vi "remoteControlTest.vi"() -> ()   [LabVIEW 2019]
uses:
  <vilib>/ReMiSYS/ReMiSYS_WSCbot-XS/SubVI/XS_F710.ctl
  <vilib>/ReMiSYS/ReMiSYS_WSCbot-XS/SubVI/XS_stick.ctl
  <vilib>/ReMiSYS/ReMiSYS_WSCbot-XS/SubVI/XS_gamepadF710.lvclass
  WSCbot_V3_Toolkit.lvlibp/WSCBOTV3_Toolkit/IO/LowLevel/PulseCounter.ctl
  <vilib>/Platform/TimedLoop/XDataNode/timing_clust.ctl
  <vilib>/Platform/TimedLoop/XDataNode/nitl_modes.ctl
  <vilib>/Platform/TimedLoop/XDataNode/wakeup.ctl
  WSCbot_V3_Toolkit.lvlibp/WSCBOTV3_Toolkit/IO/LowLevel/IO_Chanel_DIO.ctl
  <vilib>/platform/TimedLoop/XDataNode/XDataNode.xnode
  <vilib>/Platform/TimedLoop/XDataNode/XDNodeRunTimeDep.lvlib
  WSCbot_V3_Toolkit.lvlibp
panel:
  out "leftStick_Touch\nTimes":i8
  in  "High_array(mm)":dbl[](array[numeric])=[0.0, 113.0, 200.0, 300.0]
  out "Hight":i32
  out "Front/Back":bool
  out "F710 button info.rightStick":bool
  out "up":bool
  out "Car move (cm)":dbl
  out "Wheel move (cm)":dbl[](array[numeric])
  out "F710 button info.leftStick":bool
  out "F710 button info.B":bool
  out "F710 button info.X":bool
  out "F710 button info.A":bool
  out "F710 button info.Y":bool
  out "F710 button info.RB":bool
  out "F710 button info.LB":bool
  out "ini":bool
  out "reset":bool
  out "UD touch?":bool
  out "high":dbl
  out "turn touch?":bool
  out "angle":dbl
  out "speed":dbl
  out "Error Out":errorcluster
  in  "Stop Button":bool
  in  "error in (no error)":errorcluster
  in  "INPUT S/N":string="U16N121E"
  in  "VISA resource name":refnum<visa-resource-name>="USB0::0x046D::0xC21F::145C9E1C::RAW"
  out "Stop Output":bool
  out "StepmotorTarget(mm)":dbl
  out "AxisPosition":dbl
  out "SpeedArray":dbl[](array[numeric])
  out "F710":T1
  in  "maxSpeed":dbl=800.0 format="%#_13g"
  # "總高度300mm"
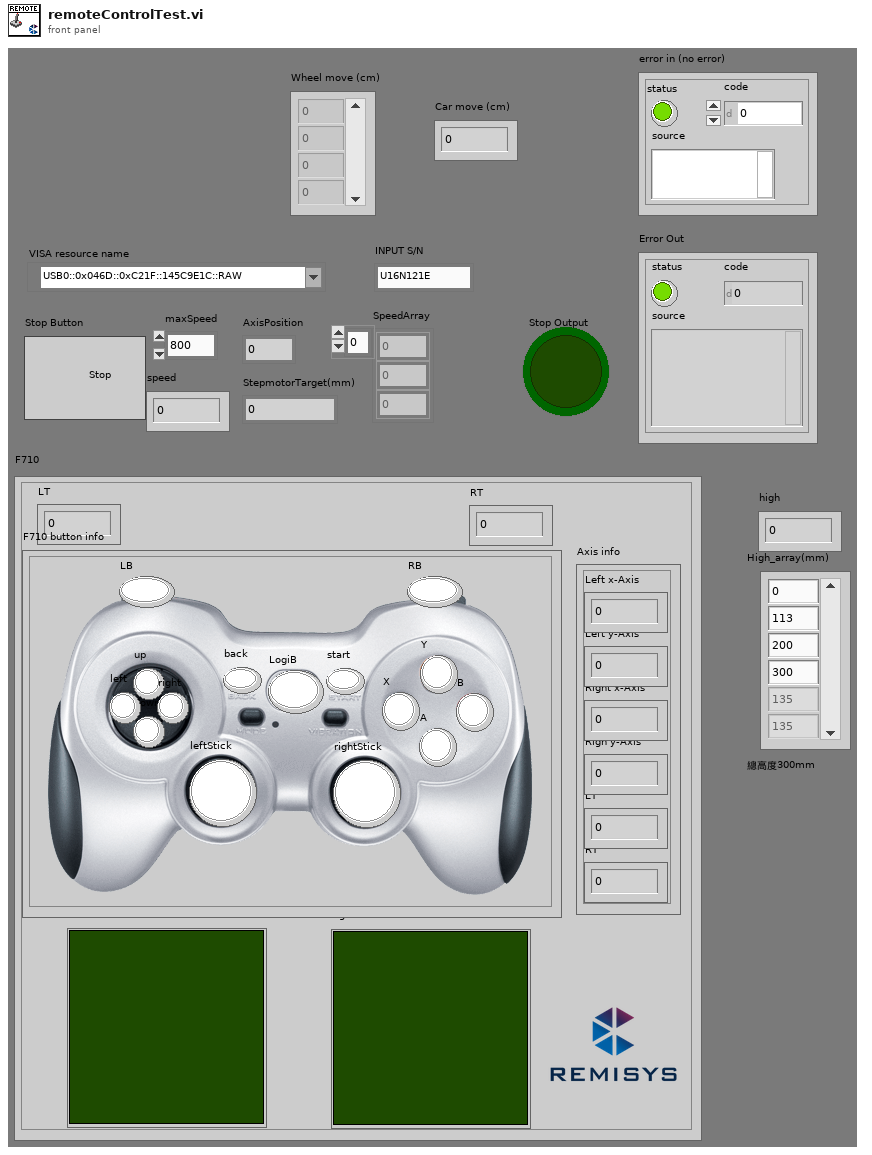
[diagram p1: front panel]
types:
  T1 = typedef "XS_F710.ctl" = cluster{"RT":u8, "LT":u8, "RightStick":T2, "LeftStick":T2, "Axis info":cluster{"Left x-Axis":i8, "Left y-Axis":i8, "Right x-Axis":i8, "Righ y-Axis":i8, "LT":u8, "RT":u8}, "F710 button info":cluster{"RB":bool, "LB":bool, "rightStick":bool, "leftStick":bool, "start":bool, "back":bool, "right":bool, "left":bool, "down":bool, "up":bool, "Y":bool, "X":bool, "B":bool, "A":bool, "LogiB":bool}}
  T2 = typedef "XS_stick.ctl" = cluster{"X":dbl, "Y":dbl}[]
  T3 = typedef "WSCbot_V3_Toolkit.lvlibp/PulseCounter.ctl" = enum16{"CH1", "CH2", "CH3", "CH4", "CH5"}
  T4 = typedef "WSCbot_V3_Toolkit.lvlibp/IO_Chanel_DIO.ctl" = enum16{"A/DIO9", "A/DIO10", "C/DIO0", "C/DIO1", "C/DIO2", "C/DIO3", "C/DIO4", "C/DIO5", "C/DIO6"}
  T5 = typedef "XDNodeRunTimeDep.lvlib/timing_clust.ctl" = cluster{"Expected End [f-1]":u64, "Actual End [f-1]":u64, "Finished Late? [f-1]":bool, "Expected End [i-1]":u64, "Actual End [i-1]":u64, "Finished Late? [i-1]":bool, "Expected Start [i]":u64, "Actual Start [i]":u64, "Expected Start [f]":u64, "Actual Start [f]":u64, "Source Name":string, "Structure Name":string, "Period":i64, "Deadline":i64, "Offset":i64, "Start":i64, "Priority":i32, "Timeout":i32, "Mode":T6, "Wakeup Reason":T7, "Error":errorcluster, "Source Type":string, "Secondary Source Type":string, "Global End Time":u64, "Global Start Time":u64, "Frame Duration":u64, "Iteration Duration":u64, "Assigned CPU":i32, "I/O Scan Engine Mode":u32}
  T6 = typedef "XDNodeRunTimeDep.lvlib/nitl_modes.ctl" = enum32{"No Change", "Process missed periods, maintain original phase", "Discard missed periods, maintain original phase", "Process missed periods, ignore original phase", "Discard missed periods, ignore original phase"}
  T7 = typedef "XDNodeRunTimeDep.lvlib/wakeup.ctl" = enum32{"Normal", "Aborted", "Asynchronous wakeup", "Timing source error", "Timed loop error", "Timeout"}
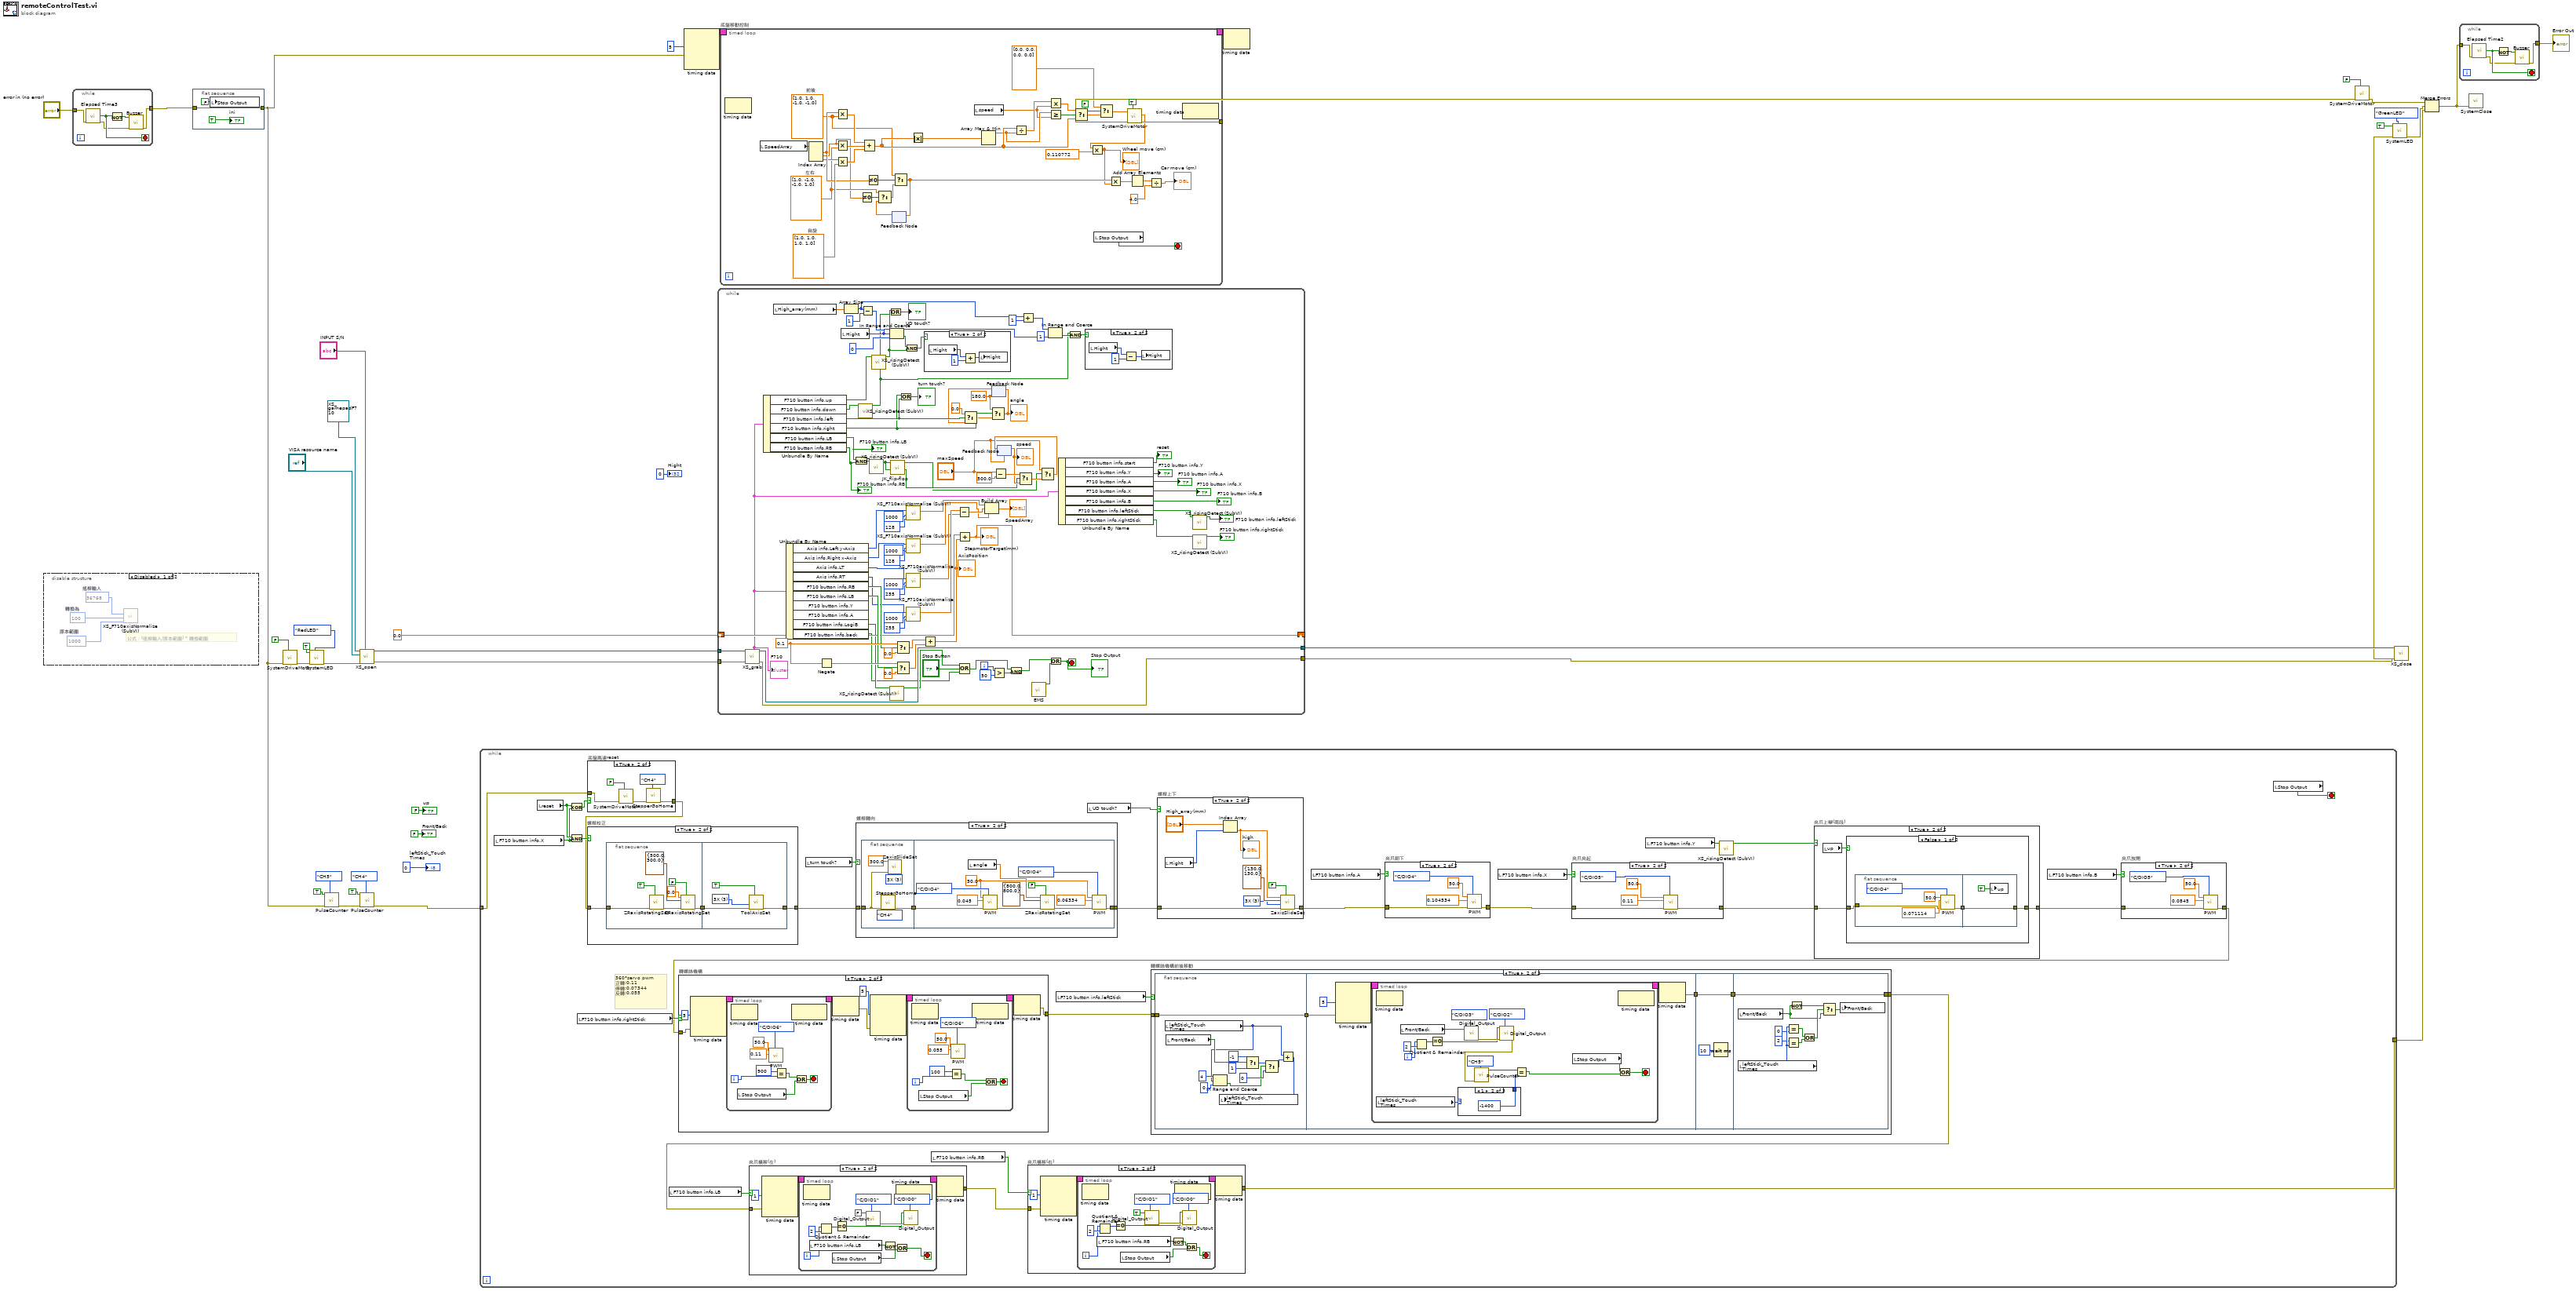
[diagram p0: block diagram]
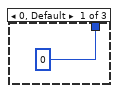
[diagram p5: hidden frame]
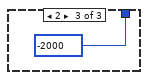
[diagram p6: hidden frame]
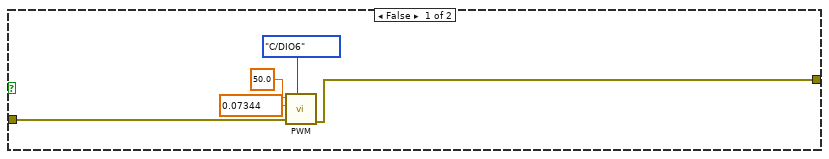
[diagram p7: hidden frame]
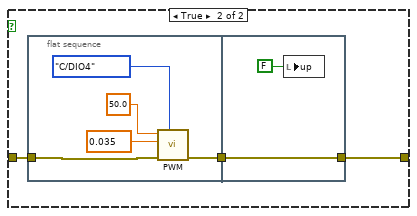
[diagram p12: hidden frame]
diagram:
  n1 = disable-structure shown="Disabled" {
    frame Disabled {
      w40 = 1000  # 原本範圍
      w41 = 100  # 轉換為
      w42 = 36768  # 搖桿輸入
      # "公式：(搖桿輸入/原本範圍) * 轉換範圍"
      n2 = call <vilib>:"XS_F710axisNormalize (SubVI).vi"("rawRange"=w40, "normalizeTo"=w41, "axisInput"=w42) -> ()  [unwired: 8 in, 1 out]
    }
    frame Enabled {
    }
  }
  n3 = while {
    tunnel: "error in (no error)" -> [w45]
    tunnel: [w43] -> w23
    stop <- w47 stop-if-true
    n4 = call "Elapsed Time3"("error in (no error)"=w45) -> ("Time has Elapsed"=w47:bool, "error out"=w44:errorcluster)  [unwired: 11 in, 6 out]
    n5 = Not(x=w47) -> (.not. x?=w46:bool)
    n6 = call "Buzzer.vi"("error in"=w44, "Set"=w46) -> ("error out"=w43:errorcluster)  [unwired: 9 in]
  }
  n7 = flat-sequence {
    tunnel: [w49] -> w7
    tunnel: w23 -> [w49]
    frame #0 {
      n8 = local write "Stop Output"(FALSE ("Stop Output")) -> ()
      "ini" <- TRUE
    }
  }
  n9 = call "SystemDriveMotor.vi"("Enable?"=FALSE, "error in"=w7) -> ("error out"=w19:errorcluster)  [unwired: 8 in, 1 out]
  n10 = call "SystemLED.vi"("SelectColor"=enum16{"RedLED", "GreenLED", "YellowLED"}."RedLED", "error in"=w19, "Set"=TRUE) -> ("error out"=w30:errorcluster)  [unwired: 8 in]
  n11 = call "PulseCounter.vi"("PulseCounterChanel"=PulseCounter."CH5", "error in"=w7, "Reset"=TRUE) -> ("error out"=w3:errorcluster)  [unwired: 7 in, 1 out]
  n12 = call <vilib>:"XS_open.vi"("INPUT S/N"="INPUT S/N", "error in (no error)"=w30, "VISA resource name"="VISA resource name", "gamepadF710 in"=refnum<class "XS_gamepadF710.lvclass"> refnum) -> ("error out"=w20:errorcluster, "gamepadF710 out"=w31:refnum<class "XS_gamepadF710.lvclass">)  [unwired: 6 in]
  n13 = call "PulseCounter.vi"("PulseCounterChanel"=PulseCounter."CH4", "error in"=w3, "Reset"=TRUE) -> ("error out"=w2:errorcluster)  [unwired: 7 in, 1 out]
  n14 = while {
    tunnel: w2 -> [w54]
    tunnel: [w57] -> w8
    stop <- w79 stop-if-true
    # "360°servo pwm\n正轉:0.11\n停轉:0.07344\n反轉:0.055"
    n15 = local read "F710 button info.X"() -> (w74:bool)
    n16 = local read "reset"() -> (w75:bool)
    n17 = Exclusive Or(1:w74, 2:w75) -> (0:w76:bool)
    n18 = And(x=w75, y=w74) -> (x .and. y?=w77:bool)
    n19 = local read "F710 button info.rightStick"() -> (w63:bool)
    n20 = case "底盤馬達reset" shown="True" w76 {
      tunnel: w54 -> [w282 w284]
      tunnel: [w282 w283] -> w53
      frame False {
      }
      frame True {
        n21 = call "SystemDriveMotor.vi"("Enable?"=FALSE, "error in"=w284) -> ("error out"=w286:errorcluster)  [unwired: 8 in, 1 out]
        n22 = call "StepperGoHome.vi"("PulseCounterChanel"=PulseCounter."CH4", "Error In"=w286) -> ("Error Out"=w283:errorcluster)  [unwired: 8 in, 1 out]
      }
    }
    n23 = case "螺桿校正" shown="True" w77 {
      tunnel: w53 -> [w288 w290]
      tunnel: [w288 w289] -> w78
      frame False {
      }
      frame True {
        n24 = flat-sequence {
          tunnel: w290 -> [w292]
          tunnel: [w296] -> w291
          tunnel: w291 -> [w302]
          tunnel: [w299] -> w289
          frame #0 {
            n25 = call "ZRaxisRotatingSet.vi"("Reset"=TRUE, "error in"=w292) -> ("error out"=w297:errorcluster)  [unwired: 8 in, 1 out]
            n26 = call "ZRaxisRotatingSet.vi"("Reset"=FALSE, "error in"=w297, "Velocity(deg/s)&ACC(deg/ss)"=cluster{"Velocity(cm/s)":dbl, "ACC(cm/ss)":dbl} {"Velocity(cm/s)"=500.0, "ACC(cm/ss)"=300.0}, "TargetHight(deg)"=0.0) -> ("error out"=w296:errorcluster)  [unwired: 6 in, 1 out]
          }
          frame #1 {
            w300 = u16 3 items=["0X", "1X", "2X", "3X"] ("findHomeVel (times)")
            n27 = call-poly "ToolAxisSet.vi"("Reset"=TRUE, "error in"=w302, "findHomeVel (times)"=w300) -> ("error out"=w299:errorcluster)  [unwired: 7 in, 1 out]
          }
        }
      }
    }
    n28 = local read "F710 button info.LB"() -> (w59:bool)
    n29 = local read "turn touch?"() -> (w52:bool)
    n30 = case "螺桿轉向" shown="True" w52 {
      tunnel: w78 -> [w312 w315]
      tunnel: [w312 w314] -> w66
      frame False {
      }
      frame True {
        n31 = flat-sequence {
          tunnel: w315 -> [w318]
          tunnel: [w320] -> w313
          tunnel: [w324] -> w314
          tunnel: w313 -> [w328]
          frame #0 {
            w316 = u16 3 items=["0X", "1X", "2X", "3X"] ("findHomeVel (times)")
            n32 = call "StepperGoHome.vi"("PulseCounterChanel"=PulseCounter."CH4", "Error In"=w318) -> ("Error Out"=w320:errorcluster)  [unwired: 8 in, 1 out]
            n33 = call "ZaxisSlideSet.vi"("error in"=w318, "findHomeVel (times)"=w316, "TargetABSHight(mm)"=300.0) -> ()  [unwired: 7 in, 2 out]
          }
          frame #1 {
            w322 = 50.0 ("Frequency(Hz)")
            n34 = local read "angle"() -> (w332:dbl)
            n35 = call "PWM.vi"("IO_Chanel"=IO_Chanel_DIO."C/DIO4", "error in"=w328, "DutyCycle"=0.045, "Frequency(Hz)"=w322) -> ("error out"=w327:errorcluster)  [unwired: 7 in]
            n36 = call "ZRaxisRotatingSet.vi"("Reset"=FALSE, "error in"=w327, "Velocity(deg/s)&ACC(deg/ss)"=cluster{"Velocity(cm/s)":dbl, "ACC(cm/ss)":dbl} {"Velocity(cm/s)"=800.0, "ACC(cm/ss)"=800.0}, "TargetHight(deg)"=w332) -> ("error out"=w325:errorcluster)  [unwired: 6 in, 1 out]
            n37 = call "PWM.vi"("IO_Chanel"=IO_Chanel_DIO."C/DIO4", "error in"=w325, "DutyCycle"=0.06334, "Frequency(Hz)"=w322) -> ("error out"=w324:errorcluster)  [unwired: 7 in]
          }
        }
      }
    }
    n38 = local read "F710 button info.RB"() -> (w56:bool)
    n39 = local read "F710 button info.leftStick"() -> (w61:bool)
    n40 = local read "UD touch?"() -> (w51:bool)
    n41 = case "螺桿上下" shown="True" w51 {
      tunnel: [w303 w309] -> w65
      tunnel: w66 -> [w303 w305]
      frame False {
      }
      frame True {
        w310 = u16 3 items=["0X", "1X", "2X", "3X"] ("findHomeVel (times)")
        n42 = local read "Hight"() -> (w304:i32)
        n43 = Index Array(array="High_array(mm)", index=w304) -> (element=w306:dbl)
        "high" <- w306
        n44 = call "ZaxisSlideSet.vi"("Reset"=FALSE, "error in"=w305, "findHomeVel (times)"=w310, "Velocity(mm/s)&ACC(mm/ss)"=cluster{"Velocity(cm/s)":dbl, "ACC(cm/ss)":dbl} {"Velocity(cm/s)"=130.0, "ACC(cm/ss)"=130.0}, "TargetABSHight(mm)"=w306) -> ("error out"=w309:errorcluster)  [unwired: 5 in, 1 out]
      }
    }
    n45 = local read "F710 button info.A"() -> (w73:bool)
    n46 = case "夾爪朝下" shown="True" w73 {
      tunnel: [w252 w254] -> w71
      tunnel: w65 -> [w252 w253]
      frame False {
      }
      frame True {
        n47 = call "PWM.vi"("IO_Chanel"=IO_Chanel_DIO."C/DIO4", "error in"=w253, "DutyCycle"=0.104534, "Frequency(Hz)"=50.0) -> ("error out"=w254:errorcluster)  [unwired: 7 in]
      }
    }
    n48 = local read "F710 button info.X"() -> (w69:bool)
    n49 = case "夾爪夾起" shown="True" w69 {
      tunnel: w71 -> [w240 w242]
      tunnel: [w240 w241] -> w64
      frame False {
      }
      frame True {
        n50 = call "PWM.vi"("IO_Chanel"=IO_Chanel_DIO."C/DIO5", "error in"=w242, "DutyCycle"=0.11, "Frequency(Hz)"=50.0) -> ("error out"=w241:errorcluster)  [unwired: 7 in]
      }
    }
    n51 = local read "F710 button info.Y"() -> (w68:bool)
    n52 = call <vilib>:"XS_risingDetect (SubVI).vi"("y"=w68) -> ("Boolean"=w67:bool)  [unwired: 10 in]
    n53 = case "夾爪上舉(兩段)" shown="True" w67 {
      tunnel: [w258 w261] -> w72
      tunnel: w64 -> [w258 w259]
      frame False {
      }
      frame True {
        n54 = local read "up"() -> (w260:bool)
        n55 = case shown="False" w260 {
          tunnel: [w264 w274] -> w261
          tunnel: w259 -> [w262 w272]
          frame False {
            n56 = flat-sequence {
              tunnel: [w267] -> w263
              tunnel: w262 -> [w265]
              tunnel: [w271] -> w264
              tunnel: w263 -> [w271]
              frame #0 {
                n57 = call "PWM.vi"("IO_Chanel"=IO_Chanel_DIO."C/DIO4", "error in"=w265, "DutyCycle"=0.071114, "Frequency(Hz)"=50.0) -> ("error out"=w267:errorcluster)  [unwired: 7 in]
              }
              frame #1 {
                n58 = local write "up"(TRUE ("up")) -> ()
              }
            }
          }
          frame True {
            n59 = flat-sequence {
              tunnel: [w276] -> w273
              tunnel: w272 -> [w275]
              tunnel: [w281] -> w274
              tunnel: w273 -> [w281]
              frame #0 {
                n60 = call "PWM.vi"("IO_Chanel"=IO_Chanel_DIO."C/DIO4", "error in"=w275, "DutyCycle"=0.035, "Frequency(Hz)"=50.0) -> ("error out"=w276:errorcluster)  [unwired: 7 in]
              }
              frame #1 {
                n61 = local write "up"(FALSE ("up")) -> ()
              }
            }
          }
        }
      }
    }
    n62 = local read "F710 button info.B"() -> (w70:bool)
    n63 = case "夾爪放開" shown="True" w70 {
      tunnel: w72 -> [w246 w248]
      tunnel: [w246 w247] -> w62
      frame False {
      }
      frame True {
        n64 = call "PWM.vi"("IO_Chanel"=IO_Chanel_DIO."C/DIO5", "error in"=w248, "DutyCycle"=0.0845, "Frequency(Hz)"=50.0) -> ("error out"=w247:errorcluster)  [unwired: 7 in]
      }
    }
    n65 = case "轉螺絲機構" shown="True" w63 {
      tunnel: w62 -> [w195 w202]
      tunnel: [w194 w200] -> w60
      frame False {
        n66 = call "PWM.vi"("IO_Chanel"=IO_Chanel_DIO."C/DIO6", "error in"=w195, "DutyCycle"=0.07344, "Frequency(Hz)"=50.0) -> ("error out"=w194:errorcluster)  [unwired: 7 in]
      }
      frame True {
        n67 = node-c288(i64 5 ("Period"), w202) -> (w207:T5)  [unwired: 2 in]
        n68 = timed-loop {
          timing: w207 -> [_]
          timing-out: [_] -> w206
          i -> [w228]
          stop <- w226 stop-if-true
          n69 = node-c288() -> ()  [unwired: 1 in, 1 out]
          n70 = local read "Stop Output"() -> (w224:bool)
          n71 = call "PWM.vi"("IO_Chanel"=IO_Chanel_DIO."C/DIO6", "DutyCycle"=0.11, "Frequency(Hz)"=50.0) -> ()  [unwired: 8 in, 1 out]
          n72 = Equal?(x=900, y=w228) -> (x = y?=w225:bool)
          n73 = node-c288() -> ()  [unwired: 1 in, 1 out]
          n74 = Or(x=w225, y=w224) -> (x .or. y?=w226:bool)
        }
        n75 = node-c288(w206) -> (w201:errorcluster)
        n76 = node-c288(i64 5 ("Period"), w201) -> (w204:T5)  [unwired: 2 in]
        n77 = timed-loop {
          timing: w204 -> [_]
          timing-out: [_] -> w203
          i -> [w212]
          stop <- w210 stop-if-true
          n78 = node-c288() -> ()  [unwired: 1 in, 1 out]
          n79 = local read "Stop Output"() -> (w208:bool)
          n80 = Equal?(x=100, y=w212) -> (x = y?=w209:bool)
          n81 = call "PWM.vi"("IO_Chanel"=IO_Chanel_DIO."C/DIO6", "DutyCycle"=0.055, "Frequency(Hz)"=50.0) -> ()  [unwired: 8 in, 1 out]
          n82 = node-c288() -> ()  [unwired: 1 in, 1 out]
          n83 = Or(x=w209, y=w208) -> (x .or. y?=w210:bool)
        }
        n84 = node-c288(w203) -> (w200:errorcluster)
      }
    }
    n85 = case "轉螺絲機構前後移動" shown="True" w61 {
      tunnel: w60 -> [w132 w137]
      tunnel: [w132 w134] -> w58
      frame False {
      }
      frame True {
        n86 = flat-sequence {
          tunnel: w137 -> [w149]
          tunnel: [w149] -> w133
          tunnel: [w150] -> w135
          tunnel: w133 -> [w151]
          tunnel: [w182] -> w136
          tunnel: w135 -> [w182]
          tunnel: [w193] -> w134
          tunnel: w136 -> [w193]
          frame #0 {
            n87 = local read "leftStick_Touch\nTimes"() -> (w139:i8)
            n88 = local read "Front/Back"() -> (w148:bool)
            n89 = In Range and Coerce(upper limit=i8 4, x=w139, lower limit=i8 0) -> (In Range?=w138:bool)  [unwired: 1 out]
            n90 = Select(t=i8 -1, s=w148, f=i8 1) -> (s? t:f=w146:i8)
            n91 = Select(t=w146, s=w138, f=i8 0) -> (s? t:f=w147:i8)
            n92 = Add(x=w139, y=w147) -> (x+y=w142:i8)
            n93 = local write "leftStick_Touch\nTimes"(w142) -> ()
          }
          frame #1 {
            n94 = node-c288(i64 5 ("Period"), w151) -> (w154:T5)  [unwired: 2 in]
            n95 = timed-loop {
              timing: w154 -> [_]
              timing-out: [_] -> w153
              i -> [w162]
              stop <- w161 stop-if-true
              n96 = node-c288() -> ()  [unwired: 1 in, 1 out]
              n97 = local read "leftStick_Touch\nTimes"() -> (w156:i8)
              n98 = local read "Front/Back"() -> (w157:bool)
              n99 = Quotient & Remainder(x=w162, y=2) -> (x-y*floor(x/y)=w166:i32)  [unwired: 1 out]
              n100 = Equal To 0?(x=w166) -> (x = 0?=w165:bool)
              n101 = case shown="1" w156 {
                tunnel: [0 ("y") -1400 ("y") -2000 ("y")] -> w159
                frame 0, Default {
                }
                frame 1 {
                }
                frame 2 {
                }
              }
              n102 = call "Digital_Output.vi"("IO_Chanel"=IO_Chanel_DIO."C/DIO3", "False/True"=w157) -> ("error out"=w169:errorcluster)  [unwired: 9 in]
              n103 = call "Digital_Output.vi"("IO_Chanel"=IO_Chanel_DIO."C/DIO2", "error in"=w169, "False/True"=w165) -> ("error out"=w163:errorcluster)  [unwired: 8 in]
              n104 = call "PulseCounter.vi"("PulseCounterChanel"=PulseCounter."CH5", "error in"=w163) -> ("PulseCount"=w158:i32)  [unwired: 8 in, 1 out]
              n105 = Equal?(x=w158, y=w159) -> (x = y?=w155:bool)
              n106 = local read "Stop Output"() -> (w160:bool)
              n107 = node-c288() -> ()  [unwired: 1 in, 1 out]
              n108 = Or(x=w160, y=w155) -> (x .or. y?=w161:bool)
            }
            n109 = node-c288(w153) -> (w150:errorcluster)
          }
          frame #2 {
            n110 = Wait (ms)(milliseconds to wait=u32 10) -> ()  [unwired: 1 out]
          }
          frame #3 {
            n111 = local read "Front/Back"() -> (w184:bool)
            n112 = local read "leftStick_Touch\nTimes"() -> (w191:i8)
            n113 = Equal?(x=w191, y=i8 0) -> (x = y?=w187:bool)
            n114 = Equal?(x=i8 2, y=w191) -> (x = y?=w188:bool)
            n115 = Not(x=w184) -> (.not. x?=w186:bool)
            n116 = Or(x=w187, y=w188) -> (x .or. y?=w185:bool)
            n117 = Select(t=w186, s=w185, f=w184) -> (s? t:f=w192:bool)
            n118 = local write "Front/Back"(w192) -> ()
          }
        }
      }
    }
    n119 = case "夾爪橫移(左)" shown="True" w59 {
      tunnel: w58 -> [w106 w108]
      tunnel: [w106 w107] -> w55
      frame False {
      }
      frame True {
        n120 = node-c288(i64 1 ("Period"), w108) -> (w111:T5)  [unwired: 2 in]
        n121 = timed-loop {
          timing: w111 -> [_]
          timing-out: [_] -> w110
          i -> [w116]
          stop <- w113 stop-if-true
          n122 = node-c288() -> ()  [unwired: 1 in, 1 out]
          n123 = local read "F710 button info.LB"() -> (w115:bool)
          n124 = Quotient & Remainder(x=w116, y=2) -> (x-y*floor(x/y)=w119:i32)  [unwired: 1 out]
          n125 = local read "Stop Output"() -> (w112:bool)
          n126 = Equal To 0?(x=w119) -> (x = 0?=w118:bool)
          n127 = call "Digital_Output.vi"("IO_Chanel"=IO_Chanel_DIO."C/DIO1", "False/True"=FALSE) -> ("error out"=w122:errorcluster)  [unwired: 9 in]
          n128 = Not(x=w115) -> (.not. x?=w114:bool)
          n129 = Or(x=w114, y=w112) -> (x .or. y?=w113:bool)
          n130 = node-c288() -> ()  [unwired: 1 in, 1 out]
          n131 = call "Digital_Output.vi"("IO_Chanel"=IO_Chanel_DIO."C/DIO0", "error in"=w122, "False/True"=w118) -> ()  [unwired: 8 in, 1 out]
        }
        n132 = node-c288(w110) -> (w107:errorcluster)
      }
    }
    n133 = case "夾爪橫移(右)" shown="True" w56 {
      tunnel: [w80 w82] -> w57
      tunnel: w55 -> [w80 w81]
      frame False {
      }
      frame True {
        n134 = node-c288(i64 1 ("Period"), w81) -> (w85:T5)  [unwired: 2 in]
        n135 = timed-loop {
          timing: w85 -> [_]
          timing-out: [_] -> w84
          i -> [w90]
          stop <- w87 stop-if-true
          n136 = node-c288() -> ()  [unwired: 1 in, 1 out]
          n137 = local read "F710 button info.RB"() -> (w89:bool)
          n138 = Quotient & Remainder(x=w90, y=2) -> (x-y*floor(x/y)=w93:i32)  [unwired: 1 out]
          n139 = Equal To 0?(x=w93) -> (x = 0?=w92:bool)
          n140 = local read "Stop Output"() -> (w86:bool)
          n141 = call "Digital_Output.vi"("IO_Chanel"=IO_Chanel_DIO."C/DIO1", "False/True"=TRUE) -> ("error out"=w96:errorcluster)  [unwired: 9 in]
          n142 = Not(x=w89) -> (.not. x?=w88:bool)
          n143 = node-c288() -> ()  [unwired: 1 in, 1 out]
          n144 = call "Digital_Output.vi"("IO_Chanel"=IO_Chanel_DIO."C/DIO0", "error in"=w96, "False/True"=w92) -> ()  [unwired: 8 in, 1 out]
          n145 = Or(x=w88, y=w86) -> (x .or. y?=w87:bool)
        }
        n146 = node-c288(w84) -> (w82:errorcluster)
      }
    }
    n147 = local read "Stop Output"() -> (w79:bool)
  }
  n148 = node-c288(i64 5 ("Period"), w7) -> (w39:T5)  [unwired: 2 in]
  n149 = while {
    tunnel: w31 -> [w424]
    tunnel: [w423] -> w35
    tunnel: [w406] -> w34
    tunnel: w20 -> [w405]
    shift-right: [w401] -> _
    shift-left: 0.0 -> [w400]
    i -> [w398]
    stop <- w364 stop-if-true
    w359 = 180.0 ("t")
    w407 = 0.1 ("t")
    n150 = call <vilib>:"XS_grab.vi"("error in (no error)"=w405, "gamepadF710 in"=w424) -> ("error out"=w406:errorcluster, "gamepadF710 out"=w423:refnum<class "XS_gamepadF710.lvclass">, "F710"=w371:T1)  [unwired: 6 in]
    "F710" <- w371
    n151 = Unbundle By Name(w371) -> ("F710 button info.up"=w352:bool, "F710 button info.down"=w337:bool, "F710 button info.left"=w356:bool, "F710 button info.right"=w355:bool, "F710 button info.LB"=w374:bool, "F710 button info.RB"=w375:bool)
    "F710 button info.LB" <- w374
    "F710 button info.RB" <- w375
    n152 = local read "High_array(mm)"() -> (w351:dbl[])
    n153 = Unbundle By Name(w371) -> ("Axis info.Left y-Axis"=w391:i8, "Axis info.Right x-Axis"=w390:i8, "Axis info.LT"=w389:u8, "Axis info.RT"=w388:u8, "F710 button info.RB"=w404:bool, "F710 button info.LB"=w403:bool, "F710 button info.LogiB"=w394:bool, "F710 button info.back"=w393:bool)  [unwired: 2 out]
    n154 = Negate(x=w407) -> (-x=w408:dbl)
    n155 = local read "Hight"() -> (w344:i32)
    n156 = Array Size(array=w351) -> (size(s)=w340:i32)
    n157 = And(x=w374, y=w375) -> (x .and. y?=w373:bool)
    n158 = call <vilib>:"XS_risingDetect (SubVI).vi"("y"=w337) -> ("Boolean"=w336:bool)  [unwired: 10 in]
    n159 = Subtract(x=w340, y=1) -> (x-y=w343:i32)
    n160 = call <vilib>:"XS_risingDetect (SubVI).vi"("y"=w373) -> ("Boolean"=w376:bool)  [unwired: 10 in]
    n161 = call <vilib>:"XS_risingDetect (SubVI).vi"("y"=w352) -> ("Boolean"=w341:bool)  [unwired: 10 in]
    n162 = Or(x=w341, y=w336) -> (x .or. y?=→"UD touch?":bool)
    n163 = In Range and Coerce(upper limit=w343, x=w344, lower limit=0) -> (In Range?=w347:bool)  [unwired: 1 out]
    n164 = call <vilib>:"XS_risingDetect (SubVI).vi"("y"=w394) -> ("Boolean"=w399:bool)  [unwired: 10 in]
    n165 = call "JK_flip-flop.vi"("K"=w376, "J"=w376) -> ("Q"=w372:bool, "-Q"=w377:bool)  [unwired: 7 in]
    n166 = Select(t=w407, s=w404, f=0.0) -> (s? t:f=w409:dbl)
    n167 = Select(t=w408, s=w403, f=0.0) -> (s? t:f=w410:dbl)
    n168 = Or(x=w355, y=w356) -> (x .or. y?=→"turn touch?":bool)
    n169 = And(x=w347, y=w341) -> (x .and. y?=w349:bool)
    n170 = call <vilib>:"XS_F710axisNormalize (SubVI).vi"("rawRange"=128, "normalizeTo"=1000, "axisInput"=w391) -> ("NormalizedValue"=w414:dbl)  [unwired: 8 in]
    n171 = call <vilib>:"XS_F710axisNormalize (SubVI).vi"("rawRange"=128, "normalizeTo"=1000, "axisInput"=w390) -> ("NormalizedValue"=w386:dbl)  [unwired: 8 in]
    n172 = call <vilib>:"XS_F710axisNormalize (SubVI).vi"("rawRange"=255, "normalizeTo"=1000, "axisInput"=w389) -> ("NormalizedValue"=w384:dbl)  [unwired: 8 in]
    n173 = call <vilib>:"XS_F710axisNormalize (SubVI).vi"("rawRange"=255, "normalizeTo"=1000, "axisInput"=w388) -> ("NormalizedValue"=w385:dbl)  [unwired: 8 in]
    n174 = Add(x=w409, y=w410) -> (x+y=w402:dbl)
    "AxisPosition" <- w402
    n175 = case shown="True" w349 {
      frame False {
      }
      frame True {
        n176 = local read "Hight"() -> (w430:i32)
        n177 = Add(x=w430, y=1) -> (x+y=w429:i32)
        n178 = local write "Hight"(w429) -> ()
      }
    }
    n179 = Subtract(x=w385, y=w384) -> (x-y=w387:dbl)
    n180 = Add(x=w400, y=w402) -> (x+y=w401:dbl)
    "StepmotorTarget(mm)" <- w401
    n181 = Compound Arithmetic op=OR(w399, "Stop Button", w393) -> (w395:bool)
    n182 = Build Array(w414, w387, w386) -> (→"SpeedArray":dbl[])
    n183 = feedback #1(w359) -> (w353:dbl)
    n184 = Select(t=0.0, s=w356, f=w353) -> (s? t:f=w354:dbl)
    n185 = Select(t=w359, s=w355, f=w354) -> (s? t:f=w358:dbl)
    "angle" <- w358
    n186 = feedback-in #1(w358) -> ()
    n187 = Greater?(x=w398, y=50) -> (0:w396:bool)
    n188 = Subtract(x="maxSpeed", y=500.0) -> (x-y=w382:dbl)
    n189 = feedback #2("maxSpeed") -> (w379:dbl)
    "speed" <- w379
    n190 = And(x=w395, y=w396) -> (x .and. y?=w365:bool)
    n191 = Select(t=w382, s=w377, f=w379) -> (s? t:f=w381:dbl)
    n192 = Add(x=w340, y=1) -> (x+y=w338:i32)
    n193 = call "EMS.vi"() -> ("EMS"=w366:bool)  [unwired: 10 in, 1 out]
    n194 = Select(t="maxSpeed", s=w372, f=w381) -> (s? t:f=w380:dbl)
    n195 = feedback-in #2(w380) -> ()
    n196 = In Range and Coerce(upper limit=w338, x=w344, lower limit=1) -> (In Range?=w345:bool)  [unwired: 1 out]
    n197 = Or(x=w365, y=w366) -> (x .or. y?=w364:bool)
    "Stop Output" <- w364
    n198 = Unbundle By Name(w371) -> ("F710 button info.start"=→"reset":bool, "F710 button info.Y"=→"F710 button info.Y":bool, "F710 button info.A"=→"F710 button info.A":bool, "F710 button info.X"=→"F710 button info.X":bool, "F710 button info.B"=→"F710 button info.B":bool, "F710 button info.leftStick"=w333:bool, "F710 button info.rightStick"=w362:bool)
    n199 = And(x=w336, y=w345) -> (x .and. y?=w348:bool)
    n200 = case shown="True" w348 {
      frame False {
      }
      frame True {
        n201 = local read "Hight"() -> (w427:i32)
        n202 = Subtract(x=w427, y=1) -> (x-y=w426:i32)
        n203 = local write "Hight"(w426) -> ()
      }
    }
    n204 = call <vilib>:"XS_risingDetect (SubVI).vi"("y"=w362) -> ("Boolean"=→"F710 button info.rightStick":bool)  [unwired: 10 in]
    n205 = call <vilib>:"XS_risingDetect (SubVI).vi"("y"=w333) -> ("Boolean"=→"F710 button info.leftStick":bool)  [unwired: 10 in]
  }
  n206 = timed-loop "底盤移動控制" {
    timing: w39 -> [_]
    timing-out: [_] -> w38
    tunnel: [w450] -> w17
    stop <- w455 stop-if-true
    w466 = dbl[] [1.0, 1.0, 1.0, 1.0]  # 自旋
    w440 = dbl[] [1.0, -1.0, -1.0, 1.0]  # 左右
    w441 = dbl[] [1.0, 1.0, -1.0, -1.0]  # 前後
    n207 = node-c288() -> ()  [unwired: 1 in, 1 out]
    n208 = local read "SpeedArray"() -> (w459:dbl[])
    n209 = Index Array(array=w459) -> (element #1=w444:dbl, element #2=w431:dbl, element #3=w442:dbl)  [unwired: 3 in]
    n210 = Multiply(x=w444, y=w441) -> (x*y=w465:dbl[])
    n211 = Multiply(x=w431, y=w440) -> (x*y=w464:dbl[])
    n212 = Multiply(x=w442, y=w466) -> (x*y=w463:dbl[])
    n213 = Not Equal To 0?(x=w431) -> (x != 0?=w443:bool)
    n214 = Compound Arithmetic op=ADD(w465, w464, w463) -> (w460:dbl[])
    n215 = Not Equal To 0?(x=w444) -> (x != 0?=w445:bool)
    n216 = feedback #3() -> (w438:dbl[])  [unwired: 1 in]
    n217 = Select(t=w440, s=w443, f=w438) -> (s? t:f=w439:dbl[])
    n218 = Select(t=w441, s=w445, f=w439) -> (s? t:f=w437:dbl[])
    n219 = feedback-in #3(w437) -> ()
    n220 = Absolute Value(x=w460) -> (abs(x)=w462:dbl[])
    n221 = local read "speed"() -> (w448:dbl)
    n222 = Array Max & Min(array=w462) -> (max value=w456:dbl)  [unwired: 3 out]
    n223 = Divide(x=w460, y=w456) -> (x/y=w458:dbl[])
    n224 = Multiply(x=w458, y=w448) -> (x*y=w457:dbl[])
    n225 = Greater Or Equal?(x=w456, y=w448) -> (x >= y?=w461:bool)
    n226 = Select(t=w457, s=w461, f=w460) -> (s? t:f=w454:dbl[])
    n227 = local read "Stop Output"() -> (w455:bool)
    n228 = Select(t=dbl[] [0.0, 0.0, 0.0, 0.0], s=FALSE, f=w454) -> (s? t:f=w452:dbl[])
    n229 = call "SystemDriveMotor.vi"("Enable?"=TRUE, "4xMotor(deg/s)"=w452) -> ("error out"=w450:errorcluster, "ENC (deg)"=w447:dbl[])  [unwired: 8 in]
    n230 = Multiply(x=w447, y=0.110772 ("Numeric")) -> (x*y=w436:dbl[])
    "Wheel move (cm)" <- w436
    n231 = Multiply(x=w437, y=w436) -> (x*y=w435:dbl[])
    n232 = Add Array Elements(numeric array=w435) -> (sum=w434:dbl)
    n233 = Divide(x=w434, y=4.0) -> (x/y=→"Car move (cm)":dbl)
    n234 = node-c288() -> ()  [unwired: 1 in, 1 out]
  }
  n235 = node-c288(w38) -> ()  [unwired: 1 out]
  n236 = call "SystemDriveMotor.vi"("Enable?"=FALSE, "error in"=w17) -> ("error out"=w16:errorcluster)  [unwired: 8 in, 1 out]
  n237 = call <vilib>:"XS_close.vi"("error in (no error)"=w34, "gamepadF710 in"=w35) -> ("error out"=w27:errorcluster)  [unwired: 8 in, 1 out]
  n238 = call "SystemLED.vi"("SelectColor"=enum16{"RedLED", "GreenLED", "YellowLED"}."GreenLED", "error in"=w27, "Set"=TRUE) -> ("error out"=w21:errorcluster)  [unwired: 8 in]
  n239 = Merge Errors(w16, w21, w8) -> (w25:errorcluster)
  n240 = while {
    tunnel: w25 -> [w471]
    tunnel: [w469] -> w10
    stop <- w473 stop-if-true
    n241 = call "Elapsed Time2"("error in (no error)"=w471) -> ("Time has Elapsed"=w473:bool, "error out"=w470:errorcluster)  [unwired: 11 in, 6 out]
    n242 = Not(x=w473) -> (.not. x?=w472:bool)
    n243 = call "Buzzer.vi"("error in"=w470, "Set"=w472) -> ("error out"=w469:errorcluster)  [unwired: 9 in]
  }
  "Error Out" <- w10
  n244 = call "SystemClose.vi"("error in"=w25) -> ()  [unwired: 2 in, 1 out]
  "Front/Back" <- FALSE ("Boolean")
  "Hight" <- 0 ("Hight")
  "up" <- FALSE ("up")
  "leftStick_Touch\nTimes" <- i8 0 ("leftStick_Touch\nTimes")
